vi "WaitUntil.vi"(7 "Time to wait until":timestamp, 9 "Skip wait on error?":bool=TRUE caption="Skip wait on error? (T)", 11 "Error in":errorcluster caption="Error in (no error)", 12 "Skip wait?":bool caption="Skip wait? (F)", 13 "Abort wait on occurrence":refnum<k4> caption="Abort wait on occurrence (none)") -> (15 "Error out":errorcluster)   [LabVIEW 2017, in "GPTiming.lvlib"]
doc: "Waits until <B>Time to wait until</B>.\n\nIf you wire an occurrence to the optional <B>Abort wait on occurrence</B> input you can abort the wait prematurely by setting that occurrence.\n\nIf <B>Time to wait until</B> is in the past this function will return immediately.\n\nThis VI is inlined. It skips the wait if there is an error on <B>Error in</B> AND <B>Skip wait on error?</B> is True (which is the default). It also skips the wait unconditionally if <B>Skip wait?</B> is True.\n\n<B>Note</B>\nThis function initially compares the current local time with the input <B>Time to wait until</B> time stamp, and then it calculates how long it has to wait. It does not adjust its wake-up time if the local time is changed while it waits. This function is capped at a maximum time to wait at around 6 years.\n\nSteen Schmidt\nGPower\n2/11 2014"
uses:
  GPTiming.lvlib
panel:
  # "Copyright © 2014\nGPower\nSee enclosed license file for terms and conditions"
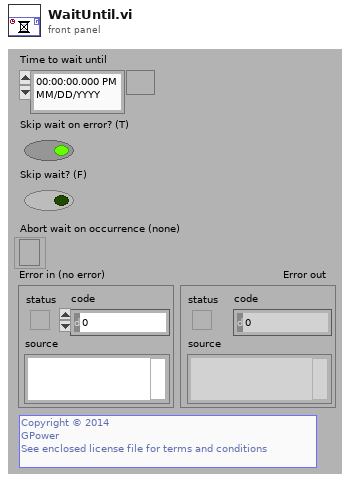
[diagram p1: front panel]
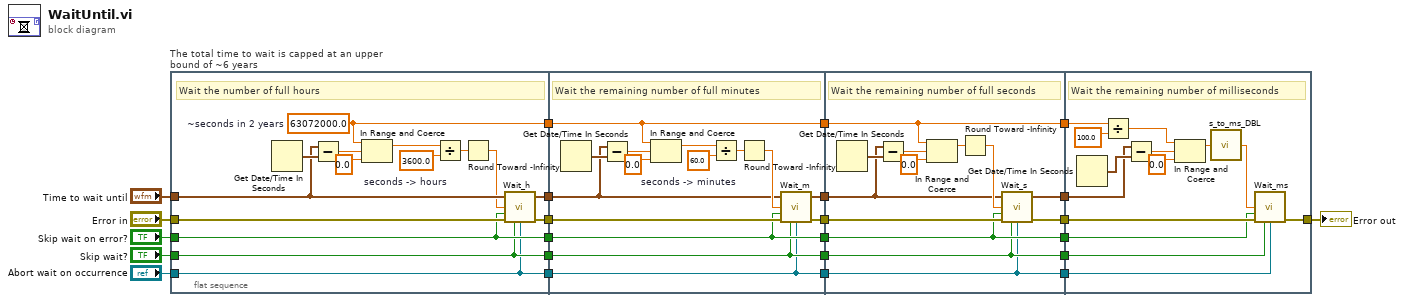
[diagram p0: block diagram]
diagram:
  n1 = flat-sequence "The total time to wait is capped at an upper bound of ~6 years" {
    tunnel: "Error in" -> [w31]
    tunnel: "Time to wait until" -> [w30]
    tunnel: [w30] -> w23
    tunnel: [w32] -> w22
    tunnel: "Skip wait on error?" -> [w28]
    tunnel: "Skip wait?" -> [w27]
    tunnel: "Abort wait on occurrence" -> [w26]
    tunnel: [w28] -> w17
    tunnel: [w27] -> w16
    tunnel: [w26] -> w15
    tunnel: [w25] -> w3
    tunnel: w23 -> [w43]
    tunnel: w22 -> [w46]
    tunnel: w17 -> [w42]
    tunnel: w16 -> [w41]
    tunnel: w15 -> [w40]
    tunnel: [w44] -> w14
    tunnel: [w43] -> w13
    tunnel: [w42] -> w12
    tunnel: [w41] -> w11
    tunnel: [w40] -> w10
    tunnel: w3 -> [w39]
    tunnel: [w39] -> w2
    tunnel: w14 -> [w64]
    tunnel: w13 -> [w57]
    tunnel: w12 -> [w56]
    tunnel: w11 -> [w55]
    tunnel: w10 -> [w54]
    tunnel: [w63] -> w9
    tunnel: [w57] -> w8
    tunnel: [w56] -> w7
    tunnel: [w55] -> w6
    tunnel: [w54] -> w5
    tunnel: w2 -> [w53]
    tunnel: [w53] -> w1
    tunnel: [w77] -> w4
    tunnel: w9 -> [w78]
    tunnel: w8 -> [w73]
    tunnel: w7 -> [w70]
    tunnel: w6 -> [w69]
    tunnel: w5 -> [w68]
    tunnel: w1 -> [w67]
    frame #0 {
      w25 = 63072000.0  # ~seconds in 2 years
      w37 = 3600.0  # seconds -> hours
      # "Wait the number of full hours"
      n2 = Get Date/Time In Seconds() -> (seconds since 1Jan1904=w33:timestamp)
      n3 = Subtract(x=w30, y=w33) -> (x-y=w34:dbl)
      n4 = In Range and Coerce(upper limit=w25, x=w34, lower limit=0.0) -> (coerced(x)=w36:dbl)  [unwired: 1 out]
      n5 = Divide(x=w36, y=w37) -> (x/y=w38:dbl)
      n6 = Round Toward -Infinity(1:w38) -> (0:w29:dbl)
      n7 = call "Wait_h.vi"("Time to wait"=w29, "Skip wait on error?"=w28, "Error in"=w31, "Skip wait?"=w27, "Abort wait on occurrence"=w26) -> ("Error out"=w32:errorcluster)  [unwired: 10 in]
    }
    frame #1 {
      w51 = 60.0  # seconds -> minutes
      # "Wait the remaining number of full minutes"
      n8 = Get Date/Time In Seconds() -> (seconds since 1Jan1904=w47:timestamp)
      n9 = Subtract(x=w43, y=w47) -> (x-y=w48:dbl)
      n10 = In Range and Coerce(upper limit=w39, x=w48, lower limit=0.0) -> (coerced(x)=w50:dbl)  [unwired: 1 out]
      n11 = Divide(x=w50, y=w51) -> (x/y=w52:dbl)
      n12 = Round Toward -Infinity(1:w52) -> (0:w45:dbl)
      n13 = call "Wait_m.vi"("Time to wait"=w45, "Skip wait on error?"=w42, "Error in"=w46, "Skip wait?"=w41, "Abort wait on occurrence"=w40) -> ("Error out"=w44:errorcluster)  [unwired: 10 in]
    }
    frame #2 {
      # "Wait the remaining number of full seconds"
      n14 = Get Date/Time In Seconds() -> (seconds since 1Jan1904=w62:timestamp)
      n15 = Subtract(x=w57, y=w62) -> (x-y=w61:dbl)
      n16 = In Range and Coerce(upper limit=w53, x=w61, lower limit=0.0) -> (coerced(x)=w59:dbl)  [unwired: 1 out]
      n17 = Round Toward -Infinity(1:w59) -> (0:w58:dbl)
      n18 = call "Wait_s.vi"("Time to wait"=w58, "Skip wait on error?"=w56, "Error in"=w64, "Skip wait?"=w55, "Abort wait on occurrence"=w54) -> ("Error out"=w63:errorcluster)  [unwired: 10 in]
    }
    frame #3 {
      # "Wait the remaining number of milliseconds"
      n19 = Get Date/Time In Seconds() -> (seconds since 1Jan1904=w74:timestamp)
      n20 = Divide(x=w67, y=100.0) -> (x/y=w66:dbl)
      n21 = Subtract(x=w73, y=w74) -> (x-y=w75:dbl)
      n22 = In Range and Coerce(upper limit=w66, x=w75, lower limit=0.0) -> (coerced(x)=w72:dbl)  [unwired: 1 out]
      n23 = call "s_to_ms_DBL.vi"("time in"=w72) -> ("time out"=w71:dbl)  [unwired: 4 in]
      n24 = call "Wait_ms.vi"("Time to wait"=w71, "Skip wait on error?"=w70, "Error in"=w78, "Skip wait?"=w69, "Abort wait on occurrence"=w68) -> ("Error out"=w77:errorcluster)  [unwired: 10 in]
    }
  }
  "Error out" <- w4
